vi "TestStage3.vi"() -> ()   [LabVIEW 2013]
uses:
  <vilib>/Utility/file.llb/Write To Spreadsheet File (DBL).vi
  <vilib>/express/express arith-compare/Formula/XNode/ExpressFormulaBlockNode.xnode
panel:
  out "iteration":dbl
  in  "speed":dbl
  out "currentPosition":dbl
  in  "Motor COM Port":refnum<visa-resource-name>="COM4"
  in  "Encoder COM Port":refnum<visa-resource-name>="COM1"
  in  "nRuns":i32
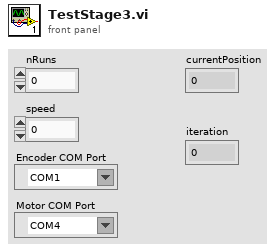
[diagram p1: front panel]
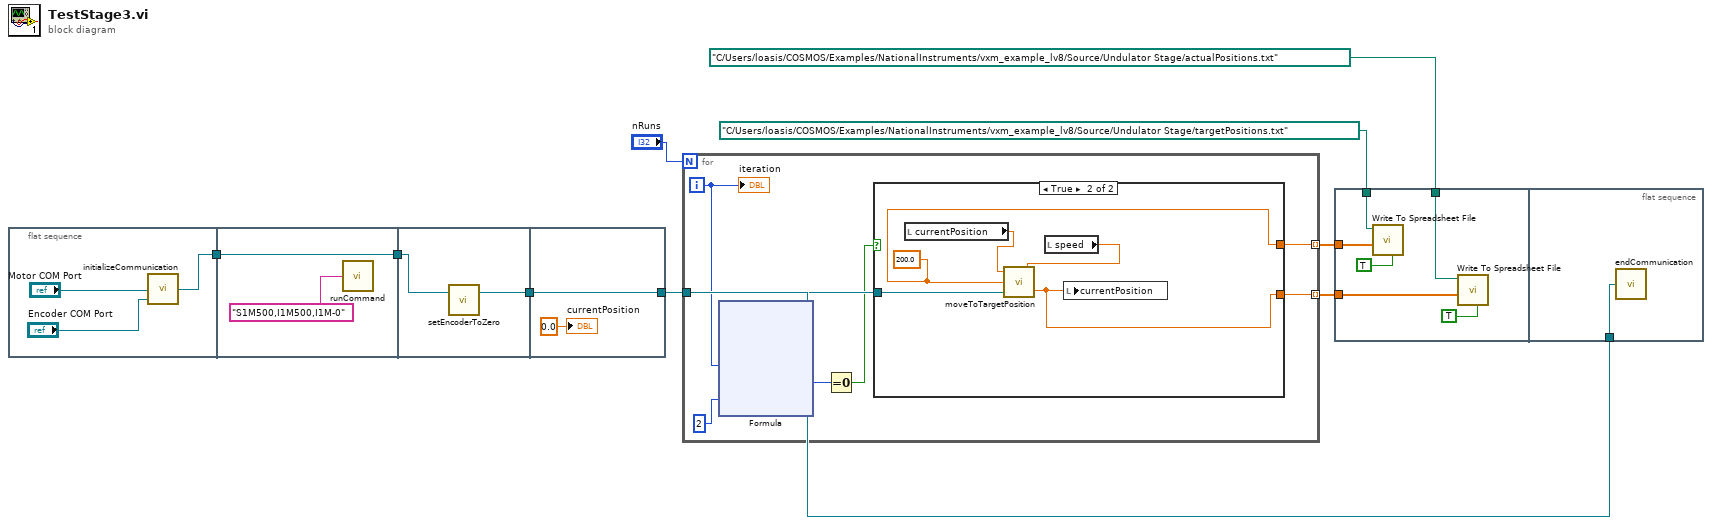
[diagram p0: block diagram]
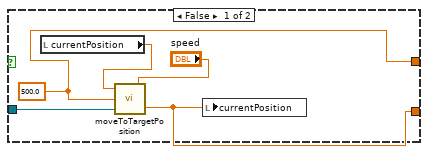
[diagram p2: hidden frame]
diagram:
  n1 = flat-sequence {
    tunnel: [w10] -> w7
    tunnel: [w13] -> w8
    tunnel: w7 -> [w13]
    tunnel: w8 -> [w16]
    tunnel: [w15] -> w6
    tunnel: [w18] -> w1
    tunnel: w6 -> [w18]
    frame #0 {
      n2 = call "initializeCommunication.vi"("Encoder COM Port"="Encoder COM Port", "Motor COM Port"="Motor COM Port") -> ("Encoder VISA Resource Name (out)"=w10:refnum<visa-resource-name>)  [unwired: 1 in]
    }
    frame #1 {
      n3 = call "runCommand.vi"("command"="S1M500,I1M500,I1M-0") -> ()  [unwired: 1 in]
    }
    frame #2 {
      n4 = call "setEncoderToZero.vi"("VISA resource name"=w16) -> ("VISA resource name out"=w15:refnum<visa-resource-name>)  [unwired: 1 in, 1 out]
    }
    frame #3 {
      "currentPosition" <- 0.0 ("currentPosition")
    }
  }
  n5 = for {
    N: "nRuns" -> [_]
    tunnel: w1 -> [w25]
    tunnel: [w24] -> w5 mode=indexing
    tunnel: [w23] -> w4 mode=indexing
    i -> [w19]
    n6 = xnode "Formula"("X1"=w19, "X2"=i8 2) -> ("Result"=w20:i32)  [unwired: 1 in, 1 out]
    n7 = Equal To 0?(x=w20) -> (x = 0?=w21:bool)
    n8 = case shown="True" w21 {
      tunnel: w25 -> [w40 w45]
      tunnel: [w37 w41] -> w23
      tunnel: [w36 w42] -> w24
      frame False {
        w36 = 500.0
        n9 = local read "currentPosition"() -> (w39:dbl)
        n10 = call "moveToTargetPosition.vi"("speed"="speed", "Encoder COM Port"=w40, "targetPos"=w36, "currentPos"=w39) -> ("updatedCurrentPos"=w37:dbl)
        n11 = local write "currentPosition"(w37) -> ()
      }
      frame True {
        w42 = 200.0
        n12 = local read "currentPosition"() -> (w44:dbl)
        n13 = local read "speed"() -> (w43:dbl)
        n14 = call "moveToTargetPosition.vi"("speed"=w43, "Encoder COM Port"=w45, "targetPos"=w42, "currentPos"=w44) -> ("updatedCurrentPos"=w41:dbl)
        n15 = local write "currentPosition"(w41) -> ()
      }
    }
    "iteration" <- w19
  }
  n16 = flat-sequence {
    tunnel: w5 -> [w51]
    tunnel: w4 -> [w50]
    tunnel: path "C:/Users/loasis/COSMOS/Examples/NationalInstruments/vxm_example_lv8/Source/Undulator Stage/targetPositions.txt" ("file path (dialog if empty)") -> [w49]
    tunnel: path "C:/Users/loasis/COSMOS/Examples/NationalInstruments/vxm_example_lv8/Source/Undulator Stage/actualPositions.txt" ("file path (dialog if empty)") -> [w48]
    tunnel: w1 -> [w52]
    frame #0 {
      n17 = call-poly <vilib>:"Write To Spreadsheet File.vi"("transpose? (no:F)"=TRUE, "1D data"=w51, "file path (dialog if empty)"=w49) -> ()  [unwired: 5 in, 1 out]
      n18 = call-poly <vilib>:"Write To Spreadsheet File.vi"("transpose? (no:F)"=TRUE, "1D data"=w50, "file path (dialog if empty)"=w48) -> ()  [unwired: 5 in, 1 out]
    }
    frame #1 {
      n19 = call "endCommunication.vi"("Encoder COM Port"=w52) -> ()  [unwired: 1 in]
    }
  }
